vi "Gain Ranging Example.vi"() -> ()   [LabVIEW 2019]
uses:
  <vilib>/Analysis/4window.llb/windowTd.ctl
  SubVIs/Low-level/TypeDefs/Resources.ctl
  <vilib>/userdefined/High Color/nirio_resource_hc.ctl
  SubVIs/Low-level/TypeDefs/Detected mmWave Adapters.ctl
  SubVIs/Low-level/TypeDefs/mmWave Adapter Information.ctl
  SubVIs/Low-level/TypeDefs/Front End Configuration.ctl
  SubVIs/Low-level/TypeDefs/Channel Configuration.ctl
  <instrlib>/niMmWave/ni3620/Config/v1/Host/Public/Typedefs/mmWave Port.ctl
  SubVIs/Low-level/TypeDefs/Hardware Configuration.ctl
  SubVIs/Low-level/TypeDefs/Direction.ctl
  SubVIs/Low-level/TypeDefs/Gain Setting.ctl
  <instrlib>/niMmWave/ni3620/Config/v1/FPGA/Public/Typedefs/TX1 RX1 Port.ctl
  SubVIs/mmWave HW Control/mmWave HW Control.lvlib
  <vilib>/Analysis/NI_AALPro.lvlib
  <instrlib>/niMmWave/ni3620/Config/v1/Host/niMmWave Config v1 Host.lvlib
panel:
  in  "indicators tab":T1(tab)=enum."Instructions"
  out "time domain":waveform(dbl)[](graph)
  out "frequency domain":cluster{"Ramp Pattern":dbl[], dbl[]}[](graph)
  in  "window":T2=8 items=["Rectangle"=0, "Hanning"=1, "Hamming"=2, "Blackman-Harris"=3, "Exact Blackman"=4, "Blackman"=5, "Flat Top"=6, "4 Term B-Harris "=7, "7 Term B-Harris"=8, "Low Sidelobe"=9, "Blackman Nuttall"=11, "Triangle"=30, "Bartlett-Hanning"=31, "Bohman"=32, "Parzen"=33, "Welch"=34, "Kaiser"=60, "Dolph-Chebyshev"=61, "Gaussian"=62]
  out "time domain power":waveform(dbl)[](graph)
  out "coerced device configuration [channel]":T3[](array[typedef]) {"Tx hardware configuration"."frequency (Hz)" format="%#_6p"; "Rx hardware configuration"."frequency (Hz)" format="%#_6p"}
  out "detected mmWave adapters [channel]":T6[](array[typedef]) {"detected mmWave adapters"."serial number" format="%.0x"}
  out "error out":errorcluster
  in  "stop":bool
  in  "controls tab":T9(tab)
  in  "option string":string="sample_rate=3.072G"
  in  "hardware resources [channel]":T10[](array[typedef])=[{"7902R (Tx)"="TxFpga0", "3610 (Tx)"="Dac0", "3620 (IF)"="IF0", "3630 (RX)"="Adc0", "7902R (Rx)"="RxFpga0"}]
  in  "hardware setup":T11
  in  "acquisition samples":u32=524288
  in  "tone frequency":dbl=500000000.0 format="%#_13p"
  in  "tone gain (dBFS)":dbl=-5.0 format="%#_13g"
  in  "device configuration [channel]":T3[](array[typedef])=[{"port select"=enum."Loopback", "Rx hardware configuration"={"gain (dB)"=20.0, "frequency (Hz)"=12000000000.0, "mmWave adapter"="None", "adapter active port"=""}, "Tx hardware configuration"={"gain (dB)"=-12.0, "frequency (Hz)"=12000000000.0, "mmWave adapter"="None", "adapter active port"=""}}] {"Tx hardware configuration"."frequency (Hz)" format="%#_6p"; "Rx hardware configuration"."frequency (Hz)" format="%#_6p"}
  in  "gain settings":fxp<+/-,16,12>[](array[numeric])=[-15.0, -20.0, -25.0, -49.0]
  in  "gain dwell time (s)":dbl=5e-05 format="%#_13p"
  in  "coarse gain values":fxp<+/-,16,12>[](array[numeric])=[-49.0, -25.0, -20.0, -15.0]
  in  "gain config triggers":string[](array[combo])=["PXI_Trig5", "PXI_Trig7"]
  in  "update gain ranging settings":bool caption="update settings"
  in  "gain ranging scope":string(combo)="tx"
  in  "gain ranging enable controls":T13={"enable fine gain ranging"=TRUE, "enable coarse gain ranging"=TRUE, "enable port config"=FALSE}
  # "Instructions:\n(1) Select device resources (Setup tab)\n(2) Select hardware setup (Setup tab)\n(3) Set device configuration\n         See datasheet for recommended gain settings\n          Warning: Incompatible gain settings may damage hardware.  \n                         Refer to datasheet for recommended gain settings.\n(4) Run this example\n\nNote: The Receiver and Transmitter must be connected (loopback) and the hardware configuration must be set\nto transceiver in order for channel equalization to occur.  When looping back at mmWave, be sure to \nconsult the datasheet to ensure sufficient path loss."
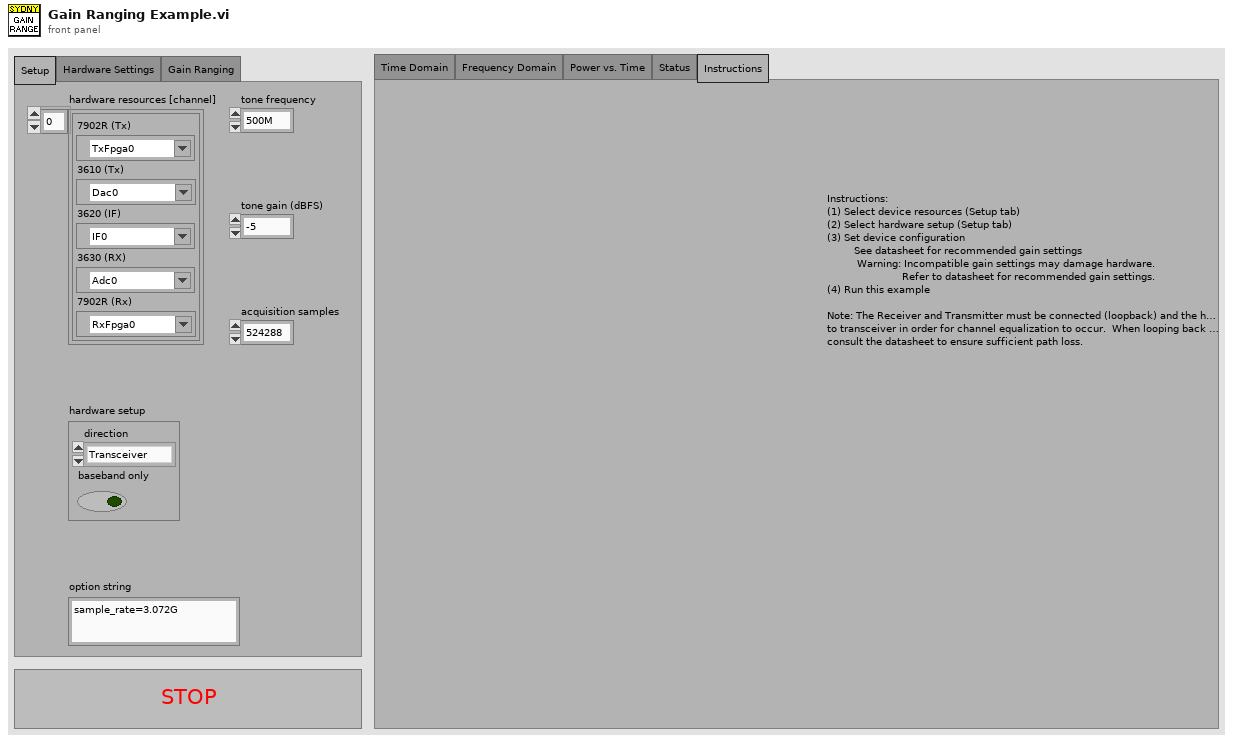
[diagram p1: front panel]
types:
  T1 = enum32{"Time Domain", "Frequency Domain", "Power vs. Time", "Status", "Instructions"}
  T2 = typedef "NI_AALPro.lvlib/windowTd.ctl" = u32
  T3 = typedef "Front End Configuration.ctl" = cluster{"port select":enum16{"IF Port", "Loopback", "Sync Port"}, "Rx hardware configuration":T4, "Tx hardware configuration":T4}
  T4 = typedef "Channel Configuration.ctl" = cluster{"gain (dB)":dbl, "frequency (Hz)":dbl, "mmWave adapter":string, "adapter active port":T5}
  T5 = typedef "niMmWave Config v1 Host.lvlib/mmWave Port.ctl" = string
  T6 = typedef "Detected mmWave Adapters.ctl" = cluster{"3620 resource name":T7, "detected mmWave adapters":T8[]}
  T7 = typedef "nirio_resource_hc.ctl" = tag
  T8 = typedef "mmWave Adapter Information.ctl" = cluster{"scope":string, "mmWave adapter type":string, "serial number":u64}
  T9 = enum32{"Setup", "Hardware Settings", "Gain Ranging"}
  T10 = typedef "Resources.ctl" = cluster{"7902R (Tx)":T7, "3610 (Tx)":refnum<visa-resource-name>, "3620 (IF)":T7, "3630 (RX)":refnum<visa-resource-name>, "7902R (Rx)":T7}
  T11 = typedef "Hardware Configuration.ctl" = cluster{"direction":T12, "baseband only":bool}
  T12 = typedef "Direction.ctl" = enum16{"Transceiver", "Receiver", "Transmitter"}
  T13 = cluster{"enable fine gain ranging":bool, "enable coarse gain ranging":bool, "enable port config":bool}
  T14 = typedef "Session.ctl" = cluster{"3620 session":refnum<queue>, "tx baseband session":T15, "rx baseband session":T23, "tx gain (dB)":dbl, "rx gain (dB)":dbl, "hardware configuration":T11, "gain ranging":T24[], "pxi trigger bus information":T25}
  T15 = typedef "Tx Baseband Session.ctl" = cluster{"3610 session":T16, "7902 reference":T22}
  T16 = typedef "ni3610_and_ni3630_Driver_Lib.lvlib/Main Settings.ctl" = cluster{"VISA resource name":refnum<visa-resource-name>, "Address Space":T17, "window_offset":u32, "register_addresses":T18, "required_MM_fpga_version":cluster{"signature":u32, "hardware":u32, "current revision":u32, "oldest revision":u32}, "CPLD Oldest Compat Version ":cluster{"hardware":u32, "CPLD firmware":u32}, "MM_FPGA_image_location":string, "is_init":bool, "card_type":T19, "DacLmkConfigFileName":string, "AdcLmkConfigFileName":string, "AdcConfigFileName":string, "DacConfigFileName_RevA":string, "DacConfigFileName_RevB":string, "Mulde hardware revision":u8, "bypass DAC PLL\n":bool, "IQ Card Revision":T20, "board capability":T21}
  T17 = typedef "VISA Register Access Address Space.ctl" = u16
  T18 = typedef "ni3610_and_ni3630_Driver_Lib.lvlib/Register Adresses.ctl" = cluster{"MM based Registers":cluster{"Revision":u32, "OldestCompatRev":u32, "signature":u32, "scratch":u32, "LedControl":u32, "BoardHwRev":u32, "BoardControl":u32, "ThermalStatus":u32, "BasebandStatus":u32, "BasebandControl":u32, "BasebandAuxSetup":u32, "BasebandAuxStatus":u32, "LmkSyncOutSetup":u32, " AdcSyncOutSetup":u32, " InjSyncOutSetup":u32, " PxiTrig0OutSetup":u32, " PxiTrig1OutSetup":u32, " PxiTrig2OutSetup":u32, " PxiTrig3OutSetup":u32, " PxiTrig4OutSetup":u32, " PxiTrig5OutSetup":u32, " PxiTrig6OutSetup":u32, " PxiTrig7OutSetup":u32}, "CPLD based Registers":cluster{"SlaveSignature":u32, "SlaveRevision":u32, "SlaveOldestCompatRev":u32, "SlaveScratch":u32, "SlaveSetup":u32, "SlaveStatus":u32, "IDacReg_offset":u32, "LMKRegGrp0_offset":u32, "QDacReg_offset":u32, "BrdTempSensorVal":u32, "TempSensorPowerDown":u32, "GPIOReg_offset":u32, "IAdcReg_offset":u32, "QAdcReg_offset":u32, "LMKRegGrp1_offset":u32, "QadcTempSensorVal":u32, "IadcTempSensorVal":u32, "RevisionReg":u32, "VcxoReg":u32, "CpldStatusReg":u32, "PowerReg":u32, "VBiasEnReg":u32, "ExtRefOeReg":u32, "QdacCtrlReg":u32, "QdacStatusReg":u32, "IdacCtrlReg":u32, "IdacStatusReg":u32, "QdacJtagIn":u32, "QdacJtagOut":u32, "IdacJtagIn":u32, "IdacJtagOut":u32, "IqDcSetupReg":u32, "QadcStatusReg":u32, "IadcStatusReg":u32, "BrdSetupReg":u32, "IqDcRevisionReg":u32, "PllStatusReg":u32, "EndpointScratchReg":u32, "AdcSyncCfgReg":u32, "IqCardOpampReg":u32}, "CPLD Register Offset":u32, "MM  Register Offset":u32, " PxiTrig0OutSetup":u32}
  T19 = typedef "ni3610_and_ni3630_Driver_Lib.lvlib/Base Card Type.ctl" = enum16{"unspecified", "ADC", "DAC"}
  T20 = typedef "ni3610_and_ni3630_Driver_Lib.lvlib/IQ Card Revision.ctl" = enum16{"RevA", "RevB", "RevC", "RevD"}
  T21 = typedef "ni3610_and_ni3630_Driver_Lib.lvlib/Board Capability.ctl" = cluster{"baseband sync":enum16{"no baseband sync", "baseband sync"}}
  T22 = typedef "Blank FPGA Reference.ctl" = refnum<k20>
  T23 = typedef "Rx Baseband Session.ctl" = cluster{"3630 session":T16, "7902 reference":T22}
  T24 = typedef "Gain Ranging.ctl" = cluster{"gain ranging active scope":string, "gain ranging stream session":refnum<k20>}
  T25 = typedef "PXI Trigger Bus Info.ctl" = cluster{"chassis resource name":refnum<visa-resource-name>, "7902R (TX)":i16, "3610 (TX)":i16, "3620 (IF)":i16, "3630 (RX)":i16, "7902R (RX)":i16}
  T26 = cluster{"frequency offset (Hz)":dbl[], "response":cdb[]}
  T27 = typedef "Gain Setting.ctl" = cluster{"gain":fxp<+/-,16,12>, "port":T28}
  T28 = typedef "TX1 RX1 Port.ctl" = enum8{"RX1", "TX1/RX2"}
  T29 = typedef "Constants.ctl" = cluster{"data clock rate (Hz)":dbl, "sample rate (Hz)":dbl, "sample rate selector string":string, "default tx bitfile path":path, "default rx bitfile path":path, "default proc bitfile path":path}
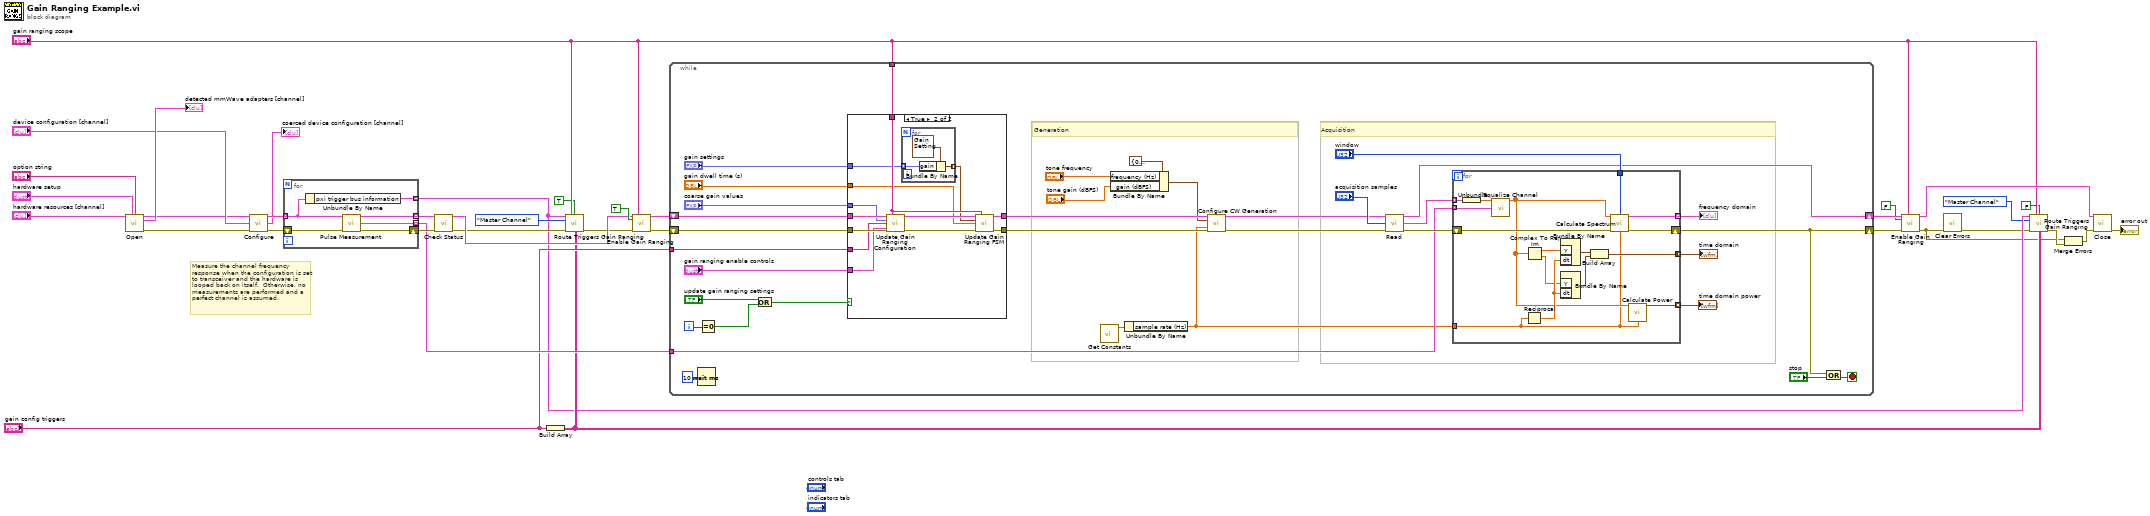
[diagram p0: block diagram]
diagram:
  # "Measure the channel frequency\nresponse when the configuration is set\nto transceiver and the hardware is \nlooped back on itself.  Otherwise, no\nmeasurements are performed and a\nperfect channel is assumed."
  n1 = call "Open.vi"("resources"="hardware resources [channel]", "hardware configuration"="hardware setup", "option string"="option string") -> ("session out"=w28:T14[], "detected mmWave adapters"=→"detected mmWave adapters [channel]":T6[], "error out"=w27:errorcluster)  [unwired: 10 in]
  n2 = call "Configure.vi"("session in"=w28, "device configuration [channel]"="device configuration [channel]", "error in"=w27) -> ("session out"=w31:T14[], "coerced device configuration [channel]"=→"coerced device configuration [channel]":T3[], "error out"=w30:errorcluster)  [unwired: 10 in]
  n3 = for {
    shift-right: [w41] -> w33
    shift-left: w30 -> [w39]
    tunnel: w31 -> [w38] mode=indexing
    tunnel: [w42] -> w32 mode=indexing
    tunnel: [w40] -> w29 mode=indexing
    tunnel: [w37] -> w8 mode=indexing
    n4 = Unbundle By Name(w38) -> ("pxi trigger bus information"=w37:T25)
    n5 = call "Pulse Measurement.vi"("session"=w38, "error in"=w39) -> ("session out"=w42:T14, "channel"=w40:T26, "error out"=w41:errorcluster)  [unwired: 11 in]
  }
  n6 = call "Check Status.vi"("session in"=w32, "error in"=w33) -> ("session out"=w16:T14[], "error out"=w11:errorcluster)  [unwired: 9 in, 3 out]
  n7 = Build Array("gain config triggers") -> (w9:string[][])
  n8 = call "Route Triggers Gain Ranging.vi"("pxi trigger bus configuration [channel]"=w8, "scope"="gain ranging scope", "map(T)/unmap(F)"=TRUE, "routing mode"=enum16{"Master Channel", "Independent Channels"}."Master Channel" ("Routing Mode"), "error in"=w11, "gain config PXI triggers [channel]"=w9) -> ("error out"=w15:errorcluster)  [unwired: 9 in]
  n9 = call "Enable Gain Ranging.vi"("session in"=w16, "scope"="gain ranging scope", "enable"=TRUE, "error in"=w15) -> ("session out"=w22:T14[], "error out"=w23:errorcluster)  [unwired: 10 in]
  n10 = while {
    shift-right: [w71] -> w26
    shift-left: w23 -> [w63]
    shift-right: [w70] -> w25
    shift-left: w22 -> [w64]
    tunnel: w29 -> [w67]
    tunnel: "gain ranging scope" -> [w56]
    tunnel: "gain config triggers" -> [w55]
    i -> [w60]
    stop <- w78 stop-if-true
    # "Generation"
    # "Acquisition"
    n11 = Wait (ms)(milliseconds to wait=u32 10) -> ()  [unwired: 1 out]
    n12 = Equal To 0?(x=w60) -> (x = 0?=w57:bool)
    n13 = Compound Arithmetic op=OR("update gain ranging settings", w57) -> (w59:bool)
    n14 = Wait (ms)(milliseconds to wait=u32 10) -> ()  [unwired: 1 out]
    n15 = case shown="True" w59 {
      tunnel: w64 -> [w80 w93]
      tunnel: w63 -> [w79 w92]
      tunnel: [w80 w87] -> w54
      tunnel: [w79 w86] -> w51
      tunnel: w56 -> [_ w84]
      tunnel: w55 -> [_ w90]
      tunnel: "coarse gain values" -> [_ w91]
      tunnel: "gain dwell time (s)" -> [_ w83]
      tunnel: "gain settings" -> [_ w82]
      tunnel: "gain ranging enable controls" -> [_ w89]
      frame False {
      }
      frame True {
        n16 = call "Update Gain Ranging Configuration.vi"("session in"=w93, "scope"=w84, "coarse gain ranging entries"=w91, "gain config PXI triggers"=w90, "error in"=w92, "enables"=w89) -> ("session out"=w88:T14[], "error out"=w85:errorcluster)  [unwired: 7 in, 1 out]
        n17 = for {
          tunnel: w82 -> [w95] mode=indexing
          tunnel: [w94] -> w81 mode=indexing
          n18 = Bundle By Name(cluster=T27 {"gain"=0.0, "port"=enum."RX1"} ("gain setting"), "gain"=w95) -> (w94:T27)
        }
        n19 = call "Update Gain Ranging FSM.vi"("session in"=w88, "scope"=w84, "gain setting list"=w81, "gain dwell time (s)"=w83, "error in"=w85) -> ("session out"=w87:T14[], "error out"=w86:errorcluster)  [unwired: 9 in]
      }
    }
    n20 = call "Get Constants.vi"() -> ("constants"=w44:T29)  [unwired: 15 in]
    n21 = Bundle By Name(cluster=cluster{"frequency (Hz)":dbl, "gain (dBFS)":dbl} {"frequency (Hz)"=0.0, "gain (dBFS)"=-3.0103} ("tone 1"), "frequency (Hz)"="tone frequency", "gain (dBFS)"="tone gain (dBFS)") -> (w47:cluster{"frequency (Hz)":dbl, "gain (dBFS)":dbl})
    n22 = Unbundle By Name(w44) -> ("sample rate (Hz)"=w43:dbl)
    n23 = call "Configure CW Generation.vi"("session in"=w54, "tone 1"=w47, "sample rate"=w43, "error in"=w51) -> ("session out"=w50:T14[], "error out"=w49:errorcluster)  [unwired: 10 in]
    n24 = call "Read.vi"("session in"=w50, "number of samples"="acquisition samples", "error in"=w49) -> ("session out"=w70:T14[], "data [channel]"=w68:cluster{"data":cdb[]}[], "error out"=w69:errorcluster)  [unwired: 10 in]
    n25 = for {
      tunnel: [w112] -> w66 mode=concatenating
      tunnel: [w111] -> w73 mode=indexing
      tunnel: "window" -> [w110]
      shift-right: [w109] -> w71
      shift-left: w69 -> [w108]
      tunnel: w68 -> [w106] mode=indexing
      tunnel: w67 -> [w105] mode=indexing
      tunnel: [w104] -> w65 mode=indexing
      tunnel: w43 -> [w97]
      n26 = Unbundle(w106) -> ("data"=w107:cdb[])
      n27 = call "Equalize Channel.vi"("input data"=w107, "channel"=w105) -> ("output data"=w100:cdb[])  [unwired: 13 in]
      n28 = Reciprocal(x=w97) -> (1/x=w102:dbl)
      n29 = Complex To Re/Im(x + iy=w100) -> (x=w103:dbl[], y=w101:dbl[])
      n30 = Bundle By Name("Y"=w103, "dt"=w102) -> (w99:waveform(dbl))  [unwired: 1 in]
      n31 = Bundle By Name("Y"=w101, "dt"=w102) -> (w98:waveform(dbl))  [unwired: 1 in]
      n32 = Build Array(w99, w98) -> (w112:waveform(dbl)[])
      n33 = call "Calculate Spectrum.vi"("input data"=w100, "window"=w110, "error in"=w108, "IQ rate"=w97) -> ("spectrum output"=w111:cluster{"Ramp Pattern":dbl[], dbl[]}, "error out"=w109:errorcluster)  [unwired: 10 in]
      n34 = call "Calculate Power.vi"("input data"=w100, "IQ rate"=w97) -> ("time domain power output"=w104:waveform(dbl))  [unwired: 13 in]
    }
    "time domain" <- w66
    "frequency domain" <- w73
    "time domain power" <- w65
    n35 = Compound Arithmetic op=OR(w71, "stop") -> (w78:bool)
  }
  n36 = call "Enable Gain Ranging.vi"("session in"=w25, "scope"="gain ranging scope", "enable"=FALSE, "error in"=w26) -> ("session out"=w24:T14[], "error out"=w3:errorcluster)  [unwired: 10 in]
  n37 = call <vilib>:"Clear Errors.vi"("error in (no error)"=w3) -> ("error out"=w2:errorcluster)  [unwired: 5 in, 1 out]
  n38 = call "Route Triggers Gain Ranging.vi"("pxi trigger bus configuration [channel]"=w8, "scope"="gain ranging scope", "map(T)/unmap(F)"=FALSE, "routing mode"=enum16{"Master Channel", "Independent Channels"}."Master Channel" ("Routing Mode"), "error in"=w2, "gain config PXI triggers [channel]"=w9) -> ("error out"=w7:errorcluster)  [unwired: 9 in]
  n39 = Merge Errors(w3, w7) -> (w6:errorcluster)
  n40 = call "Close.vi"("session"=w24, "error in"=w6) -> ("error out"=→"error out":errorcluster)  [unwired: 13 in]
